vi "SVA 4MV5 PR004 CCSA RPJ SLJC.vi"() -> ()   [LabVIEW 2021]
uses:
  <vilib>/userDefined/High Color/IMAQdx.ctl
  <vilib>/picture/picture.llb/Draw True-Color Pixmap.vi
  <vilib>/vision/driver/NI_Vision_Acquisition_Software.lvlib
  <vilib>/vision/NI_Vision_Development_Module.lvlib
panel:
  out "new picture":picture
  out "output cluster":T1
  out "Image":T2(plugin-control)
  in  "Detener \nprograma":bool
  in  "Session In":T3
  # "Práctica 4: Momentos invariantes de Hu \nIntegrantes:\nCUEVAS CERÓN SERGIO ALBERTO\nREYES PÉREZ JAVIER\nSALCEDO LICEA JUAN CARLOS"
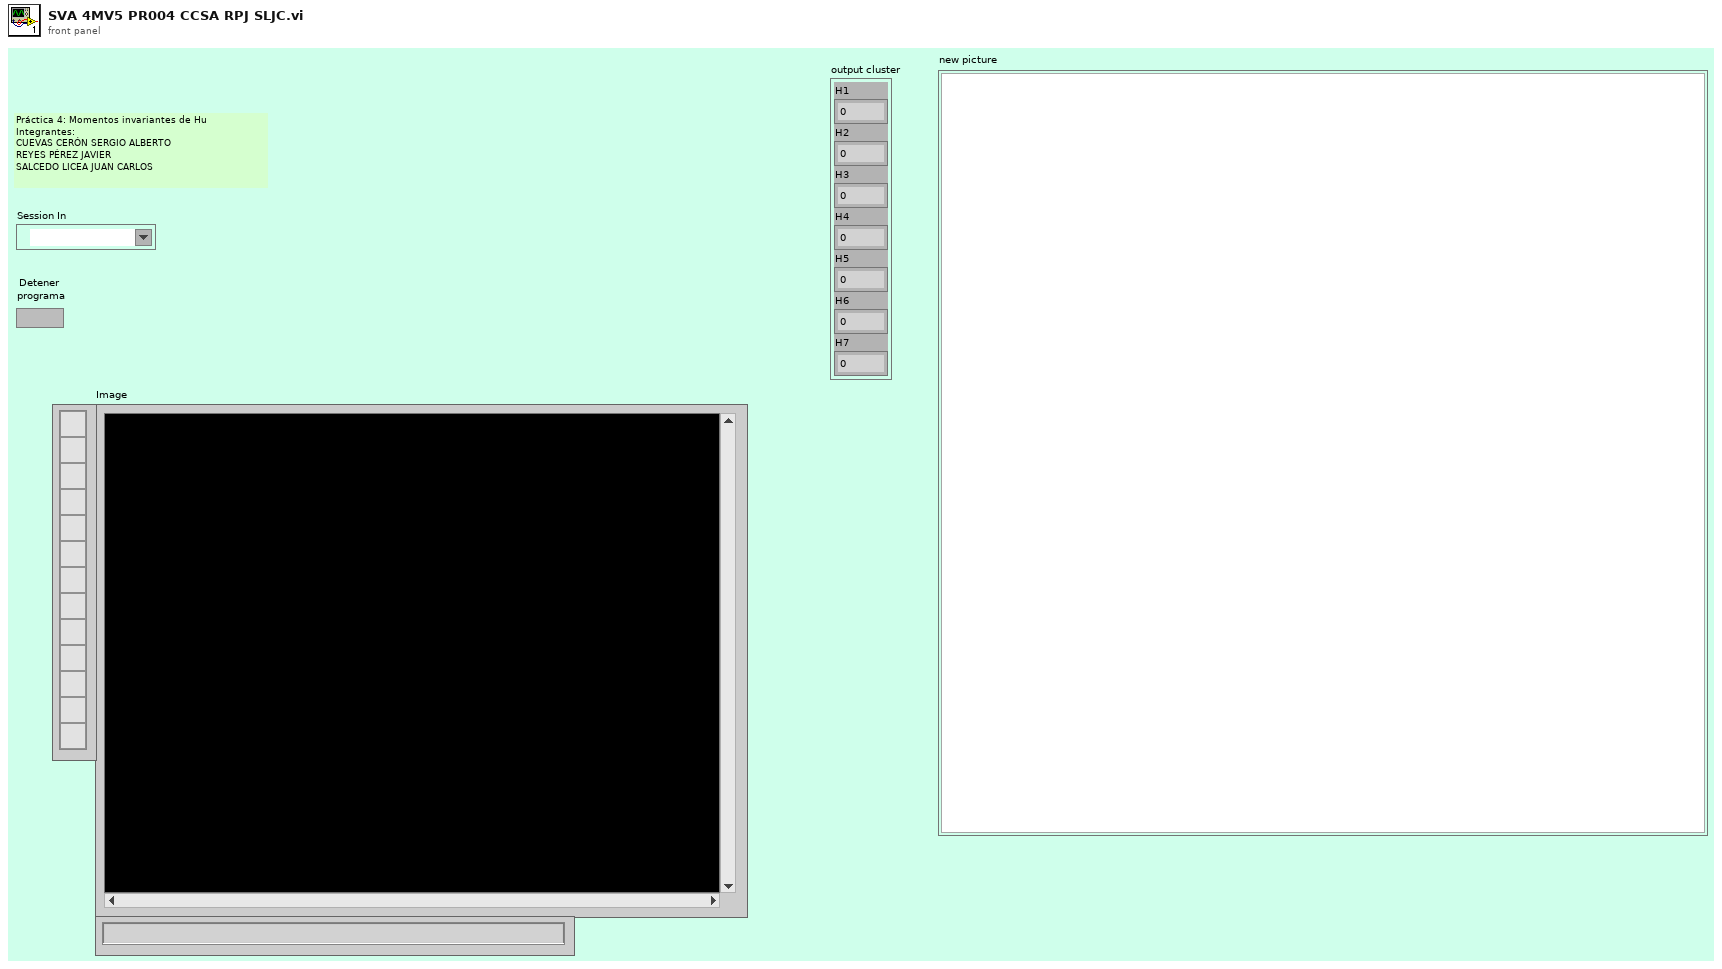
[diagram p1: front panel]
types:
  T1 = cluster{"H1":dbl, "H2":dbl, "H3":dbl, "H4":dbl, "H5":dbl, "H6":dbl, "H7":dbl}
  T2 = typedef "IMAQ Image.ctl" = refnum<image>
  T3 = typedef "IMAQdx.ctl" = refnum<k21>
  T4 = typedef "Image Type" = u32
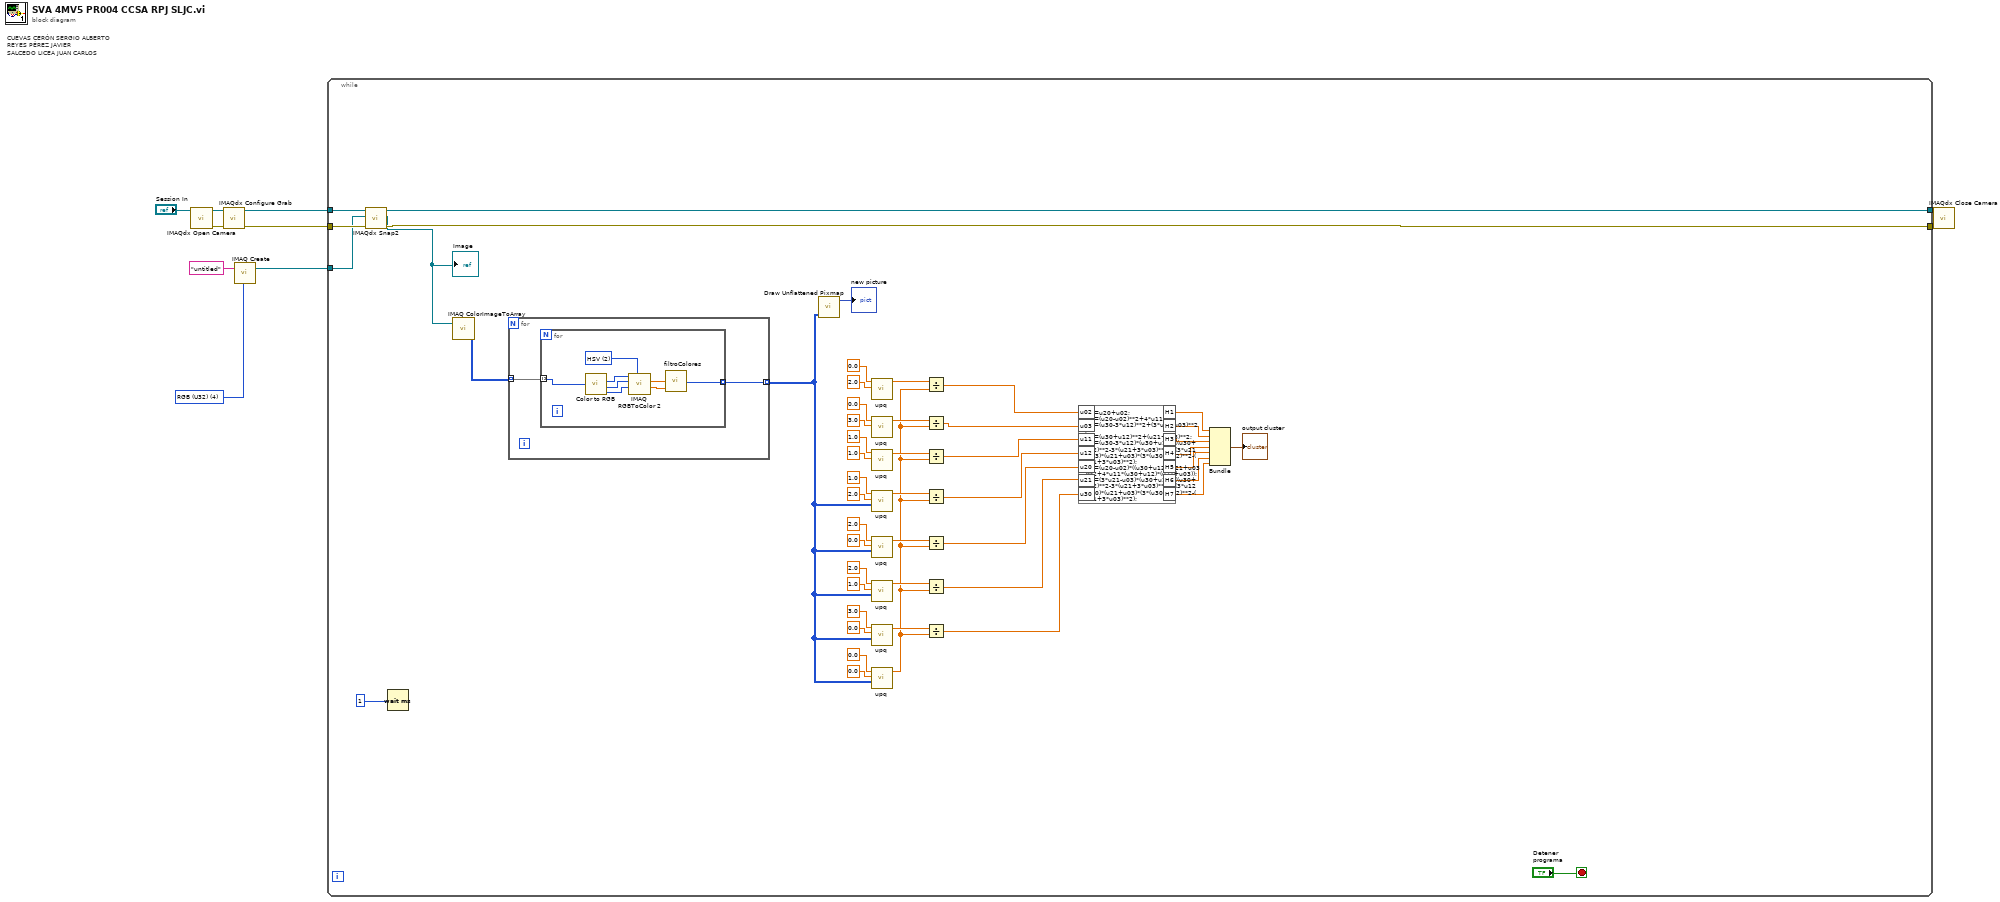
[diagram p0: block diagram]
diagram:
  w9 = T4 4 items=["Grayscale (U8)", "Grayscale (I16)", "Grayscale (SGL)", "Complex (CSG)", "RGB (U32)", "HSL (U32)", "RGB (U64)", "Grayscale (U16)"] ("Image Type")
  # "CUEVAS CERÓN SERGIO ALBERTO\nREYES PÉREZ JAVIER\nSALCEDO LICEA JUAN CARLOS"
  n1 = call <vilib>:"IMAQdx Open Camera.vi"("Session In"="Session In") -> ("error out"=w7:errorcluster, "Session Out"=w6:T3)  [unwired: 9 in]
  n2 = call <vilib>:"IMAQdx Configure Grab.vi"("error in"=w7, "Session In"=w6) -> ("error out"=w4:errorcluster, "Session Out"=w5:T3)  [unwired: 8 in]
  n3 = call "IMAQ Create"("Image Name"="untitled", "Image Type"=w9) -> ("New Image"=w1:T2)  [unwired: 3 in, 1 out]
  n4 = while {
    tunnel: w5 -> [w59]
    tunnel: w4 -> [w58]
    tunnel: [w57] -> w3
    tunnel: [w56] -> w2
    tunnel: w1 -> [w54]
    stop <- "Detener \nprograma" stop-if-true
    n5 = call <vilib>:"IMAQdx Snap2.vi"("error in"=w58, "Image In"=w54, "Session In"=w59) -> ("error out"=w56:errorcluster, "Image Out"=w53:T2, "Session Out"=w57:T3)  [unwired: 6 in]
    "Image" <- w53
    n6 = Wait (ms)(milliseconds to wait=u32 1) -> ()  [unwired: 1 out]
    n7 = call "IMAQ ColorImageToArray"("Image"=w53) -> ("Image Pixels (U32)"=w52:u32[][])  [unwired: 3 in, 2 out]
    n8 = for {
      tunnel: w52 -> [w62] mode=indexing
      tunnel: [w61] -> w32 mode=indexing
      n9 = for {
        tunnel: w62 -> [w66] mode=indexing
        tunnel: [w63] -> w61 mode=indexing
        w67 = u16 2 items=["RGB", "HSL", "HSV", "HSI", "CIE L*a*b*", "CIE XYZ"] ("Color Mode")
        n10 = call <vilib>:"Color to RGB.vi"("Color"=w66) -> ("R"=w70:u8, "G"=w69:u8, "B"=w68:u8)  [unwired: 1 out]
        n11 = call "IMAQ RGBToColor 2"("Color Mode"=w67, "Blue value"=w68, "Green value"=w69, "Red value"=w70) -> ("Blue or Luma or Val or Inten or Z or b*value"=w65:dbl, "Green or Sat or Y or a* value"=w64:dbl)  [unwired: 4 in, 2 out]
        n12 = call "filtroColores.vi"("V"=w65, "S"=w64) -> ("Color"=w63:u32)  [unwired: 2 in, 1 out]
      }
    }
    n13 = call-poly <vilib>:"Draw Unflattened Pixmap.vi"("data (RGB format)"=w32) -> ("new picture"=→"new picture":picture)  [unwired: 8 in]
    n14 = call "upq.vi"("q"=2.0, "p"=0.0) -> ("upq"=w24:dbl)  [unwired: 9 in]
    n15 = call "upq.vi"("q"=3.0, "p"=0.0) -> ("upq"=w23:dbl)  [unwired: 9 in]
    n16 = call "upq.vi"("q"=1.0, "p"=1.0) -> ("upq"=w19:dbl)  [unwired: 9 in]
    n17 = call "upq.vi"("ImagenBinaria"=w32, "q"=2.0, "p"=1.0) -> ("upq"=w31:dbl)  [unwired: 8 in]
    n18 = call "upq.vi"("ImagenBinaria"=w32, "q"=0.0, "p"=2.0) -> ("upq"=w22:dbl)  [unwired: 8 in]
    n19 = call "upq.vi"("ImagenBinaria"=w32, "q"=1.0, "p"=2.0) -> ("upq"=w21:dbl)  [unwired: 8 in]
    n20 = call "upq.vi"("ImagenBinaria"=w32, "q"=0.0, "p"=3.0) -> ("upq"=w20:dbl)  [unwired: 8 in]
    n21 = call "upq.vi"("ImagenBinaria"=w32, "q"=0.0, "p"=0.0) -> ("upq"=w18:dbl)  [unwired: 8 in]
    n22 = Divide(x=w24, y=w18) -> (x/y=w17:dbl)
    n23 = Divide(x=w23, y=w18) -> (x/y=w16:dbl)
    n24 = Divide(x=w19, y=w18) -> (x/y=w15:dbl)
    n25 = Divide(x=w31, y=w18) -> (x/y=w14:dbl)
    n26 = Divide(x=w22, y=w18) -> (x/y=w13:dbl)
    n27 = Divide(x=w21, y=w18) -> (x/y=w12:dbl)
    n28 = Divide(x=w20, y=w18) -> (x/y=w11:dbl)
    n29 = formula code="H1=u20+u02;\nH2=(u20-u02)**2+4*u11;\nH3=(u30-3*u12)**2+(3*u21-u03)**2;\nH4=(u30+u12)**2+(u21+u03)**2;\nH5=(u30-3*u12)*(u30+u12)*((u30+u12)**2-3*(u21+3*u03)**2)+(3*u21-u03)*(u21+u03)*(3*(u30+u12)**2-(u21+3*u03)**2);\nH6=(u20-u02)*((u30+u12)-(u21+u03)**2+4*u11*(u30+u12)*(u21+u03));\nH7=(3*u21-u03)*(u30+u12)*((u30+u12)**2-3*(u21+3*u03)**2)+(3*u12-u30)*(u21+u03)*(3*(u30+u12)**2-(u21+3*u03)**2);"("u02"=w17, "u03"=w16, "u11"=w15, "u12"=w14, "u20"=w13, "u21"=w12, "u30"=w11) -> ("H1"=w43:dbl, "H2"=w44:dbl, "H3"=w45:dbl, "H4"=w46:dbl, "H5"=w47:dbl, "H6"=w48:dbl, "H7"=w49:dbl)
    n30 = Bundle("H1"=w43, "H2"=w44, "H3"=w45, "H4"=w46, "H5"=w47, "H6"=w48, "H7"=w49) -> (→"output cluster":T1)  [unwired: 1 in]
  }
  n31 = call <vilib>:"IMAQdx Close Camera.vi"("error in"=w2, "Session In"=w3) -> ()  [unwired: 9 in, 1 out]
